vi "setSaveImages.vi"(8 "error in (no error)":errorcluster, 10 "saveImages":bool, 11 "CamaraSettings in":refnum<class "CamaraSettings.lvclass">) -> (0 "error out":errorcluster, 3 "CamaraSettings out":refnum<class "CamaraSettings.lvclass">)   [LabVIEW 2011, in "Tools.lvlib" / "Settings.lvlib" / "CamaraSettings.lvclass"]
uses:
  CamaraSettings.lvclass
  CamaraSettings.lvclass/CamaraSettings.ctl
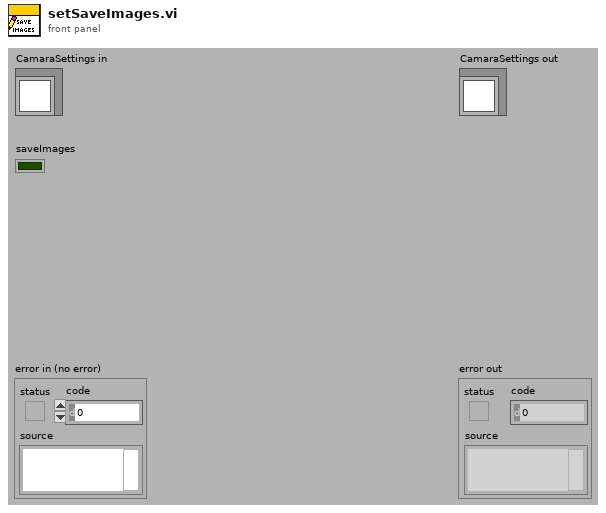
[diagram p1: front panel]
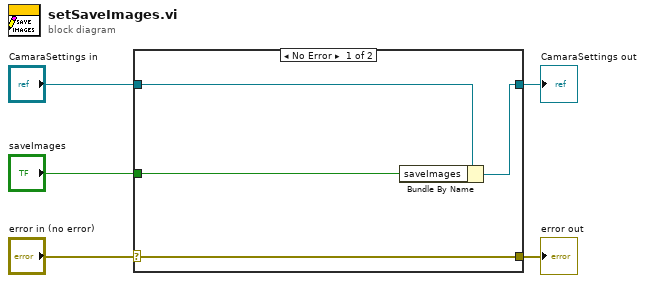
[diagram p0: block diagram]
diagram:
  n1 = case shown="No Error" "error in (no error)" {
    selector: "error in (no error)" -> [w9 w10]
    tunnel: [w9 w10] -> w4
    tunnel: [w7 w11] -> w2
    tunnel: "CamaraSettings in" -> [w8 w11]
    tunnel: "saveImages" -> [w6 _]
    frame No Error {
      n2 = Bundle By Name(cluster=w8, "saveImages"=w6) -> (w7:refnum<class "CamaraSettings.lvclass">)
    }
    frame Error {
    }
  }
  "error out" <- w4
  "CamaraSettings out" <- w2
